vi "AddMessage.vi"(0 "Message queue":refnum<queue>, 5 "Message":string, 7 "Data":variant, 9 "Message Priority ?":bool, 11 "entrée d'erreur (pas d'erreur)":errorcluster) -> (4 "Dup Message queue":refnum<queue>, 15 "error out":errorcluster)   [LabVIEW 2013, in "MessageQueues.lvlib"]
doc: "Ce VI ajoute un message avec une donnée dans une pile (message queue).\nEntrée :\n- Message Queue : Pile d'entrée\n- Message : le message \n- Data : la donnée en variant\n- Priority : Vrai => le message est mis en début de pile\nfaux => le message est mis en fin de pile.\n\nSortie :\n- Dup Message Queue : Pile incrémentée\n- error : Cluster de sortie d'erreur."
uses:
  MessageQueues.lvlib
  Message Cluster.ctl
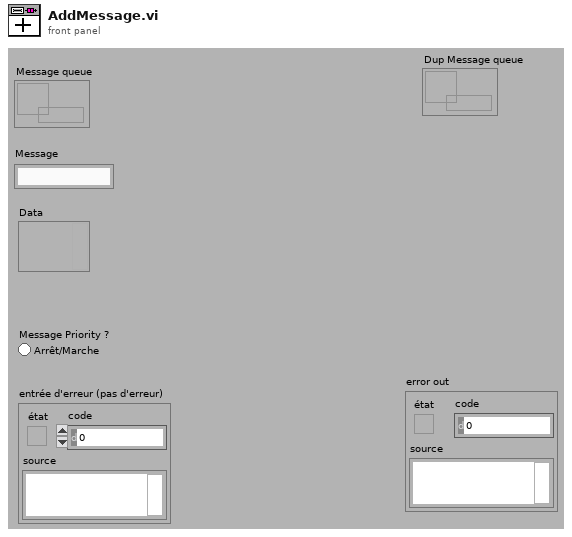
[diagram p1: front panel]
types:
  T1 = typedef "MessageQueues.lvlib/Message Cluster.ctl" = cluster{"Message":string, "Data":variant}
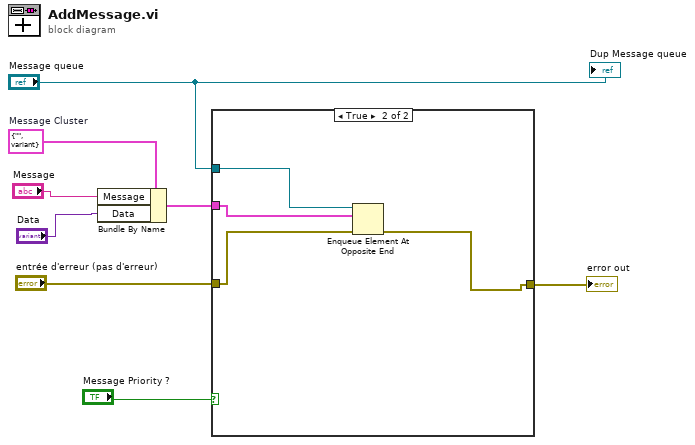
[diagram p0: block diagram]
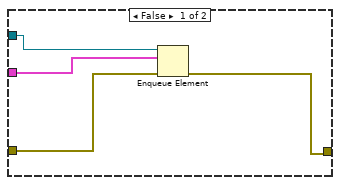
[diagram p2: hidden frame]
diagram:
  w7 = T1 {"Message"="", "Data"=variant}  # Message Cluster
  n1 = Bundle By Name(cluster=w7, "Message"="Message", "Data"="Data") -> (w4:T1)
  n2 = case shown="True" "Message Priority ?" {
    tunnel: w4 -> [w12 w13]
    tunnel: "Message queue" -> [w11 w14]
    tunnel: "entrée d'erreur (pas d'erreur)" -> [w10 w16]
    tunnel: [w9 w15] -> w1
    frame False {
      n3 = Enqueue Element(queue=w11, element=w12, error in (no error)=w10) -> (error out=w9:errorcluster)  [unwired: 1 in, 2 out]
    }
    frame True {
      n4 = Enqueue Element At Opposite End(queue=w14, element=w13, error in (no error)=w16) -> (error out=w15:errorcluster)  [unwired: 1 in, 2 out]
    }
  }
  "error out" <- w1
  "Dup Message queue" <- "Message queue"
